vi "AllowDrag.vi"(10 "DragPosition":i32, 11 "OrderSelection in":refnum<class "OrderSelection.lvclass">) -> (2 "AllowDrag?":bool, 3 "OrderSelection out":refnum<class "OrderSelection.lvclass">)   [LabVIEW 2015, in "OrderSelection.lvclass"]
uses:
  OrderSelection.lvclass
  <vilib>/Utility/miscctls.llb/LVPointTypeDef.ctl
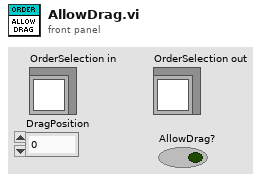
[diagram p1: front panel]
types:
  T1 = typedef "LVPointTypeDef.ctl" = cluster{"Horizontal":i16, "Vertical":i16}
  T2 = typedef "LVBoundsTypeDef.ctl" = cluster{"Width":u32, "Height":u32}
  T3 = typedef "LVRectTypeDef.ctl" = cluster{"Left":i16, "Top":i16, "Right":i16, "Bottom":i16}
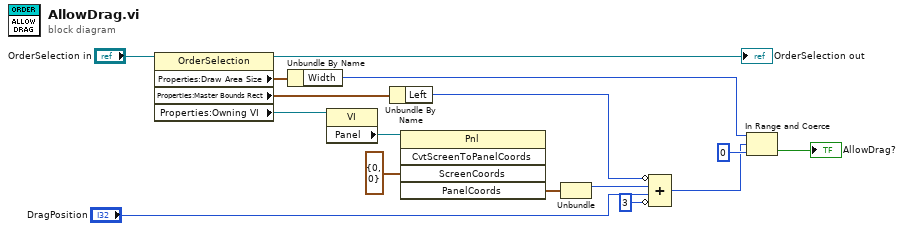
[diagram p0: block diagram]
diagram:
  n1 = property class="OrderSelection"(reference="OrderSelection in") -> (reference out=→"OrderSelection out":refnum<class "OrderSelection.lvclass">, "Properties:Draw Area Size"=w12:T2, "Properties:Master Bounds Rect"=w5:T3, "Properties:Owning VI"=w4:refnum<vi>)  [unwired: 1 in, 1 out]
  n2 = Unbundle By Name(w12) -> ("Width"=w3:u32)
  n3 = property class="VI"(reference=w4) -> ("Panel"=w6:refnum<vi>)  [unwired: 1 in, 2 out]
  n4 = Unbundle By Name(w5) -> ("Left"=w11:i16)
  n5 = invoke class="Pnl" method="CvtScreenToPanelCoords"(reference=w6, "ScreenCoords"=T1 {"Horizontal"=0, "Vertical"=0} ("Screen Coordinates")) -> ("PanelCoords"=w8:T1)  [unwired: 3 in, 4 out]
  n6 = Unbundle(w8) -> ("Horizontal"=w9:i16)  [unwired: 1 out]
  n7 = Compound Arithmetic op=ADD(invert w11, w9, "DragPosition", invert 3 ("value")) -> (w1:i32)
  n8 = In Range and Coerce(upper limit=w3, x=w1, lower limit=u32 0) -> (In Range?=→"AllowDrag?":bool)  [unwired: 1 out]
